vi "PV ActiveLine - OffsetDisplay (TPG361).vi"(7 "W/R":bool, 8 "Fehler (Eingang)":errorcluster, 10 "Sensor 1 Set":dbl format="%.4e", 11 "Referenz in":refnum<visa-resource-name>) -> (0 "Cluster (Ausgang)":errorcluster, 2 "Sensor 1 Get":dbl format="%.4e", 3 "Referenz out":refnum<visa-resource-name>)   [LabVIEW 2013, in "PV ActiveLine.lvlib"]
doc: "OFD - Offset Display (Linear Gauges)\n\nTransmit: OFD [,sa.aaaaEsaa]\nReceive: sa.aaaaEsaa\n\nsa.aaaaEsaa Gauge 1 Offset, [in current pressure unit]\n(default = 0.0000E+00)\n\nValues can be entered in any format. They are internally converted into the floating point format."
uses:
  <instrlib>/PV ActiveLine/PV ActiveLine.lvlib
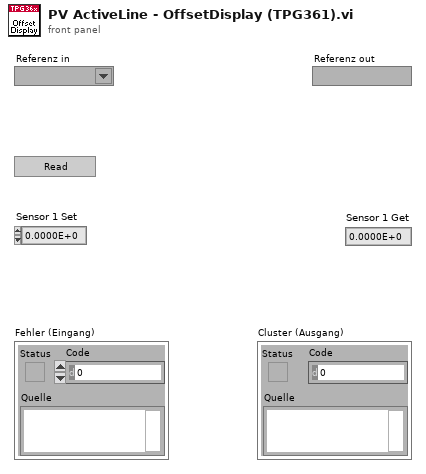
[diagram p1: front panel]
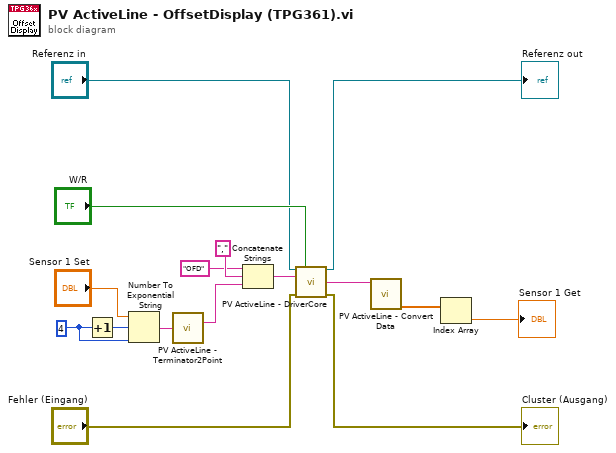
[diagram p0: block diagram]
diagram:
  w7 = u8 4 ("Kommastellen")
  n1 = Increment(x=w7) -> (x+1=w9:u8)
  n2 = Number To Exponential String(number="Sensor 1 Set", precision (6)=w7, 3:w9) -> (E-format string=w11:string)  [unwired: 1 in]
  n3 = call <instrlib>:"PV ActiveLine - Terminator2Point.vi"("Eingangstring"=w11) -> ("Ausgangstring"=w10:string)
  n4 = Concatenate Strings("OFD" ("Command"), ",", w10) -> (w4:string)
  n5 = call <instrlib>:"PV ActiveLine - DriverCore.vi"("Referenz in"="Referenz in", "Write/Read"="W/R", "Command"=w4, "Fehler (Eingang)"="Fehler (Eingang)") -> ("Referenz out"=→"Referenz out":refnum<visa-resource-name>, "String Out"=w3:string, "Cluster (Ausgang)"=→"Cluster (Ausgang)":errorcluster)  [unwired: 9 in]
  n6 = call <instrlib>:"PV ActiveLine - Convert Data.vi"("String in"=w3) -> ("DBL out"=w2:dbl[])  [unwired: 7 in, 3 out]
  n7 = Index Array(array=w2) -> (element=→"Sensor 1 Get":dbl)  [unwired: 1 in]
